vi "ROI_def_2.vi"(11 "read image/take pic":bool=TRUE) -> (0 "data_folder":path, 1 "Cal_Image path":path, 2 "Cal_Image":T1(plugin-control), 3 "ROI Descriptor":T2 {"Contours"."Type" items=["No Selection", "Point", "Line", "Rectangle", "Oval", "Polygon", "Free", "Annulus", "Unused2", "Unused3", "Broken Line", "Free Hand Line", "Rotated Rectangle"]})   [LabVIEW 2017]
uses:
  <vilib>/vision/NI_Vision_Development_Module.lvlib
panel:
  in  "ROI Image source":u16(ring) items=["constant", "take pic", "read image"]
  out "Global Rectangle":i32[](array[numeric])
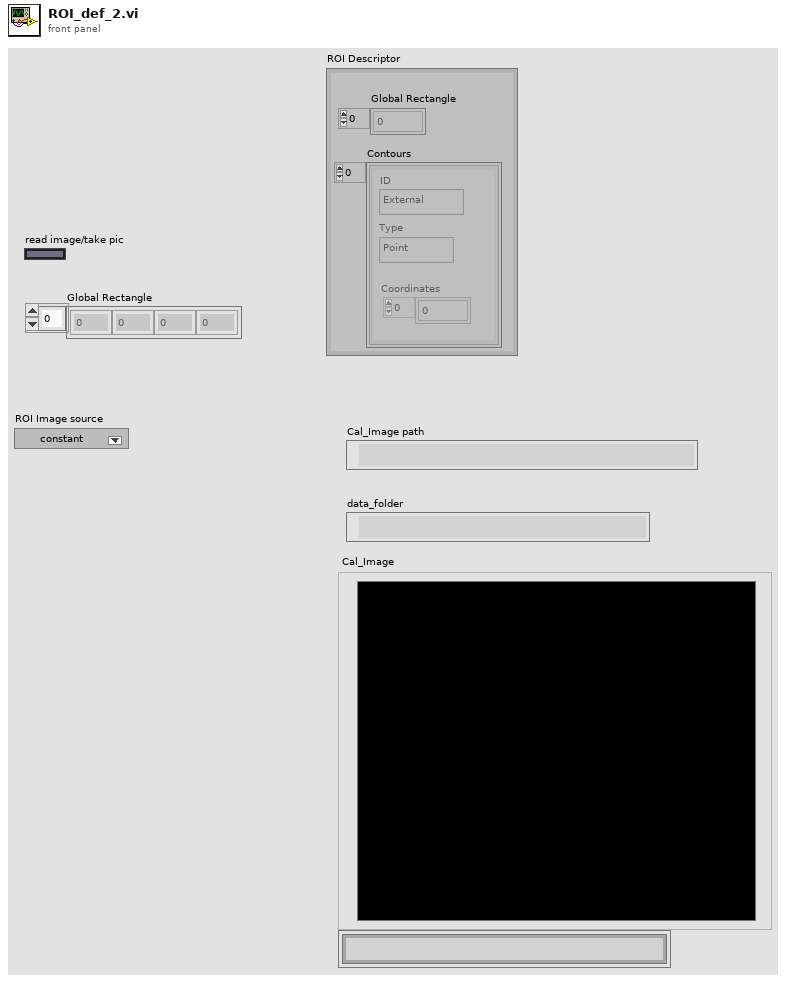
[diagram p1: front panel]
types:
  T1 = typedef "IMAQ Image.ctl" = refnum<image>
  T2 = cluster{"Global Rectangle":i32[], "Contours":cluster{"ID":enum32{"External", "Internal"}, "Type":u32, "Coordinates":i32[]}[]}
  T3 = typedef "Image Type" = u32
  T4 = typedef "ROI Descriptor" = cluster{"Global Rectangle":i32[], "Contours":cluster{"ID":enum32{"External", "Internal"}, "Type":u32, "Coordinates":i32[]}[]}
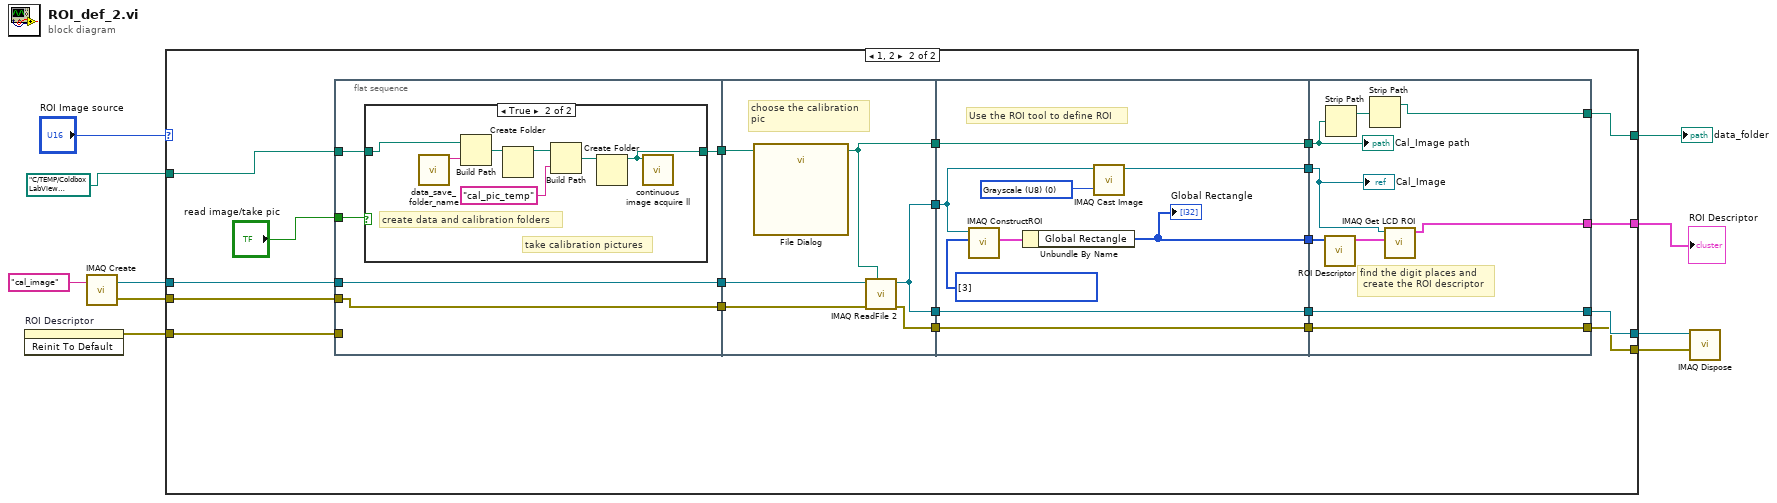
[diagram p0: block diagram]
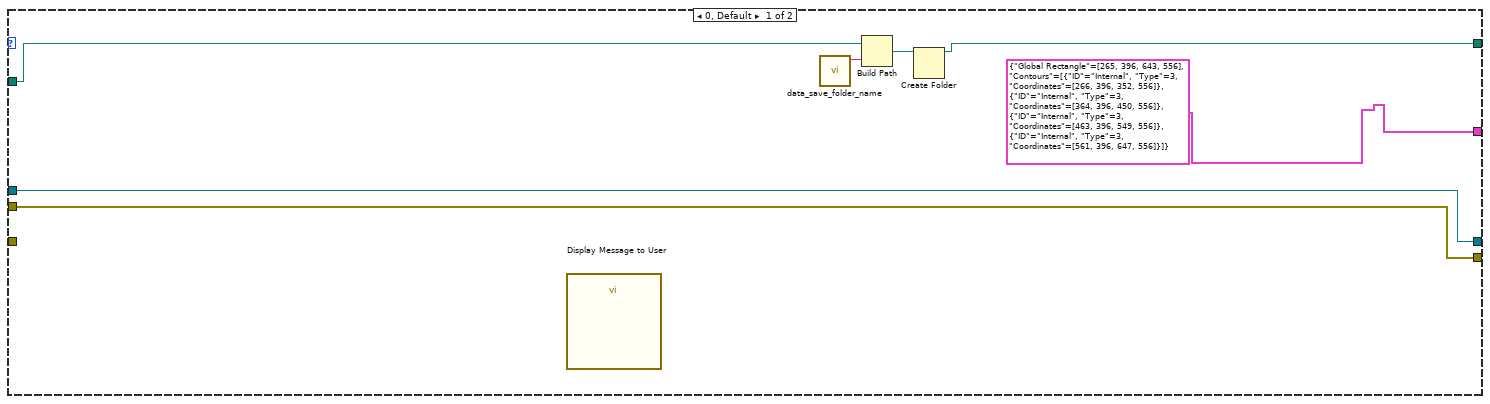
[diagram p2: hidden frame]
diagram:
  n1 = invoke on="ROI Descriptor" class="Clust (strict)" method="Reinit To Default"() -> (error out=w8:errorcluster)  [unwired: 3 in, 2 out]
  n2 = call "IMAQ Create"("Image Name"="cal_image") -> ("New Image"=w2:T1, "error out"=w1:errorcluster)  [unwired: 4 in]
  n3 = case shown="1, 2" "ROI Image source" {
    tunnel: [w17 w27] -> w10
    tunnel: [w16 w26] -> w9
    tunnel: w8 -> [_ w25]
    tunnel: [w12 w24] -> w7
    tunnel: [T2 {"Global Rectangle"=[265, 396, 643, 556], "Contours"=[{"ID"=enum."Internal", "Type"=3, "Coordinates"=[266, 396, 352, 556]}, {"ID"=enum."Internal", "Type"=3, "Coordinates"=[364, 396, 450, 556]}, {"ID"=enum."Internal", "Type"=3, "Coordinates"=[463, 396, 549, 556]}, {"ID"=enum."Internal", "Type"=3, "Coordinates"=[561, 396, 647, 556]}]} ("ROI Descriptor") w23] -> w5
    tunnel: path "C:/TEMP/Coldbox LabView Development/calib" ("Data/Calib folder 2") -> [w14 w22]
    tunnel: w2 -> [w17 w20]
    tunnel: w1 -> [w16 w19]
    frame 0, Default {
      n4 = call "Display Message to User"() -> ()  [unwired: 10 in, 2 out]
      n5 = call "data_save_folder_name.vi"() -> ("concatenated string"=w15:string)  [unwired: 11 in]
      n6 = Build Path(base path=w14, name or relative path=w15) -> (appended path=w13:path)
      n7 = Create Folder(path (use dialog)=w13) -> (created path=w12:path)  [unwired: 2 in, 2 out]
    }
    frame 1, 2 {
      n8 = flat-sequence {
        tunnel: "read image/take pic" -> [w39]
        tunnel: [w43] -> w38
        tunnel: w25 -> [_]
        tunnel: w22 -> [w42]
        tunnel: [w41] -> w21
        tunnel: w20 -> [w41]
        tunnel: w19 -> [w40]
        tunnel: [w40] -> w18
        tunnel: w38 -> [w57]
        tunnel: [w55] -> w37
        tunnel: [w56] -> w36
        tunnel: [w55] -> w35
        tunnel: [w54] -> w34
        tunnel: w21 -> [w53]
        tunnel: w18 -> [w52]
        tunnel: w37 -> [w63]
        tunnel: w36 -> [w58]
        tunnel: [w64] -> w33
        tunnel: [w62] -> w32
        tunnel: [w60] -> w31
        tunnel: w35 -> [w60]
        tunnel: [w59] -> w30
        tunnel: w34 -> [w59]
        tunnel: [w58] -> w29
        tunnel: w33 -> [w75]
        tunnel: w32 -> [w69]
        tunnel: w31 -> [w73]
        tunnel: w30 -> [w72]
        tunnel: [w73] -> w27
        tunnel: [w72] -> w26
        tunnel: w29 -> [w71]
        tunnel: [w68] -> w24
        tunnel: [w67] -> w23
        frame #0 {
          n9 = case shown="True" w39 {
            tunnel: [w44 w45] -> w43
            tunnel: w42 -> [w44 w46]
            frame False {
              # "read the base path for calibrtion image"
            }
            frame True {
              # "take calibration pictures"
              # "create data and calibration folders"
              n10 = call "data_save_folder_name.vi"() -> ("concatenated string"=w48:string)  [unwired: 11 in]
              n11 = Build Path(base path=w46, name or relative path=w48) -> (appended path=w49:path)
              n12 = Create Folder(path (use dialog)=w49) -> (created path=w51:path)  [unwired: 2 in, 2 out]
              n13 = Build Path(base path=w51, name or relative path="cal_pic_temp") -> (appended path=w50:path)
              n14 = Create Folder(path (use dialog)=w50) -> (created path=w45:path)  [unwired: 2 in, 2 out]
              n15 = call "continuous image acquire ll.vi"("File Path"=w45) -> ()  [unwired: 11 in]
            }
          }
        }
        frame #1 {
          # "choose the calibration\npic"
          n16 = call "File Dialog"("start path"=w57) -> ("selected path"=w56:path)  [unwired: 11 in, 3 out]
          n17 = call "IMAQ ReadFile 2"("File Path"=w56, "error in (no error)"=w52, "Image"=w53) -> ("error out"=w54:errorcluster, "Image Out"=w55:T1)  [unwired: 4 in, 3 out]
        }
        frame #2 {
          w61 = T3 0 items=["Grayscale (U8)", "Grayscale (I16)", "Grayscale (SGL)", "Complex (CSG)", "RGB (U32)", "HSL (U32)", "RGB (U64)", "Grayscale (U16)"] ("Image Type")
          w65 = u32[] [3] items=["No Selection", "Point", "Line", "Rectangle", "Oval", "Polygon", "Freehand Region", "Annulus", "Zoom", "Pan", "Broken Line", "Freehand Line", "Rotated Rectangle"] ("Tools")
          # "Use the ROI tool to define ROI"
          n18 = call "IMAQ ConstructROI"("Tools"=w65, "Image"=w63) -> ("ROI Descriptor Out"=w66:T4)  [unwired: 6 in, 3 out]
          n19 = Unbundle By Name(w66) -> ("Global Rectangle"=w64:i32[])
          "Global Rectangle" <- w64
          n20 = call "IMAQ Cast Image"("Image Type"=w61, "Image Src"=w63) -> ("Image Dst Out"=w62:T1)  [unwired: 8 in, 1 out]
        }
        frame #3 {
          # "find the digit places and\n create the ROI descriptor"
          n21 = call "ROI Descriptor.vi"("Global Rectangle"=w75) -> ("ROI Descriptor"=w74:T2)  [unwired: 10 in]
          n22 = Strip Path(path=w71) -> (stripped path=w70:path)  [unwired: 1 out]
          n23 = Strip Path(path=w70) -> (stripped path=w68:path)  [unwired: 1 out]
          n24 = call "IMAQ Get LCD ROI"("ROI Descriptor"=w74, "Image"=w69) -> ("ROI Descriptor out"=w67:T2)  [unwired: 3 in, 6 out]
          "Cal_Image path" <- w71
          "Cal_Image" <- w69
        }
      }
    }
  }
  "data_folder" <- w7
  "ROI Descriptor" <- w5
  n25 = call "IMAQ Dispose"("Image"=w10, "error in (no error)"=w9) -> ()  [unwired: 4 in, 1 out]
